vi "APC_9056_DynoControl.vi"(1 "LoadIni?":bool, 2 "PC_ControlSettings":T1={"Spark advance [CADBTDC]"=0.0, "Pref"=0.0, "O2ref"=0.0, "DI advance [CADBTDC]"=0.0, "DI duration [ms] "=0.0, "CO2ref"=0.0, "PFI duration [ms]"=0.0, "IMEP ref"=0.0, "Speed ref"=0.0, "IGN enable"=TRUE, "DI enable"=TRUE, "CL PFI\n lambda"=TRUE, "CL PFI\nIMEP"=FALSE, "Activate\ncylinder"=[FALSE, FALSE, FALSE, FALSE, FALSE, FALSE], "Force idling"=FALSE, "Force motoring"=FALSE, "ETP resync"=FALSE, "Requested mode"=0, "Clear Sync Errors"=FALSE, "toggle TDC"=FALSE, "l ref"=0.0, "PID control references"={"NG"=FALSE, "Ar"=FALSE, "O2"=FALSE, "Intake vent"=FALSE, "Cross vent"=FALSE, "Exhaust vent"=FALSE, "NG control mode"=0, "NG-FC-001-REF"=0.0, "WF-OA-002-REF"=0.0, "IMEP-REF"=0.0, "Nm-REF"=0.0, "Ar control mode"=0, "AR-PC-002-REF"=0.0, "WF-PT-004-REF"=0.0, "O2 control mode"=0, "O2-FC-001-REF"=0.0, "WF-OA-001-REF"=0.0, "Tcoolant control  mode"=0, "EC-FC-001-REF"=0.0, "EC-TT-001-REF"=0.0, "Texh control mode"=0, "SW-FC-004-REF"=0.0, "SW-FT-002-REF"=0.0, "WF-TT-004-REF"=0.0, "Toil control mode"=0, "SW-FC-009-REF"=0.0, "SW-FT-004-REF"=0.0, "EO-TT-001-REF"=0.0, "AIC201_CO2_ConcTarget"=0.0, "O2_FF_NG"=FALSE, "Dyno control mode"=0, "Membrane control mode"=0, "AR-FT-001-REF"=0.0, "MTR modbus floats"=[0.0, 0.0, 0.0, 0.0, 0.0, 0.0, 0.0, 0.0, 0.0, 0.0, 0.0, 0.0, 0.0, 0.0, 0.0, 0.0, 0.0, 0.0, 0.0], "MTR modbus u16"=[0, 0, 0, 0, 0, 0, 0], "MTR HB"=FALSE, "PC_HB"=FALSE, "EMERGENCY STOP"=FALSE}, "CA50setpoint [CADATDC]"=0.0, "CA50 control"=TRUE, "Knock control"=TRUE, "CLEAR EMERGENCY STOP"=FALSE, "EMERGENCY STOP"=FALSE}, 3 "input cluster":T3) -> (0 "DYNO-REF":dbl format="%.2f")   [LabVIEW 2020]
uses:
  controls/APC_PIDCluster.ctl
  controls/APC_ControlSettings.ctl
  controls/APC_PIDcontrolSettings.ctl
  controls/APC_cascadePIDsettings.ctl
  <vilib>/addons/control/pid/pid.llb/PID Advanced (DBL).vi
  <vilib>/Utility/xml.llb/Read From XML File(string).vi
  <vilib>/Utility/xml.llb/Write to XML File(string).vi
  <vilib>/addons/control/pid/NI_PID_pid.lvlib
panel:
  out "direct?":bool
  out "Direct control":dbl format="%.2f"
  in  "SpeedReference (manual)":dbl
  in  "save":bool
  in  "load":bool
  out "Dyno control mode":u8
  out "EngineSpeed":dbl=2293.506542256783
  in  "FF control":dbl format="%.2f"
  in  "reinitialize? (F)":bool
  in  "SpeedSetpointForPID (manual)":dbl
  in  "Dyno control mode":u8=1
  in  "PID gains":T4={"proportional gain (Kc)"=1.0, "integral time (Ti, min)"=0.01, "derivative time (Td, min)"=0.0} {"derivative time (Td, min)" format="%.3f"; "integral time (Ti, min)" format="%.3f"; "proportional gain (Kc)" format="%.3f"}
  in  "PID setpoint range":cluster{"setpoint high":dbl, "setpoint low":dbl}={"setpoint high"=100.0, "setpoint low"=0.0} {"setpoint high" format="%.2f"; "setpoint low" format="%.2f"}
  in  "PID output range":cluster{"output high":dbl, "output low":dbl}={"output high"=100.0, "output low"=-100.0} {"output low" format="%.2f"; "output high" format="%.2f"}
  in  "Override PC PID references":bool
  in  "Safe mode control":dbl format="%.2f"
  in  "learn?":bool
  out "CL on?":bool
  out "setpoint":dbl format="%.2f"
  # "Dyno control"
  # "Modes:\n0 : safe. 0 sent to dyno\n1 (default) : speed reference sent to dyno\n2 : a PID correction is added to the direct control. Tune the parameters with care (mostly slow integral action, no proportional or feed forward)"
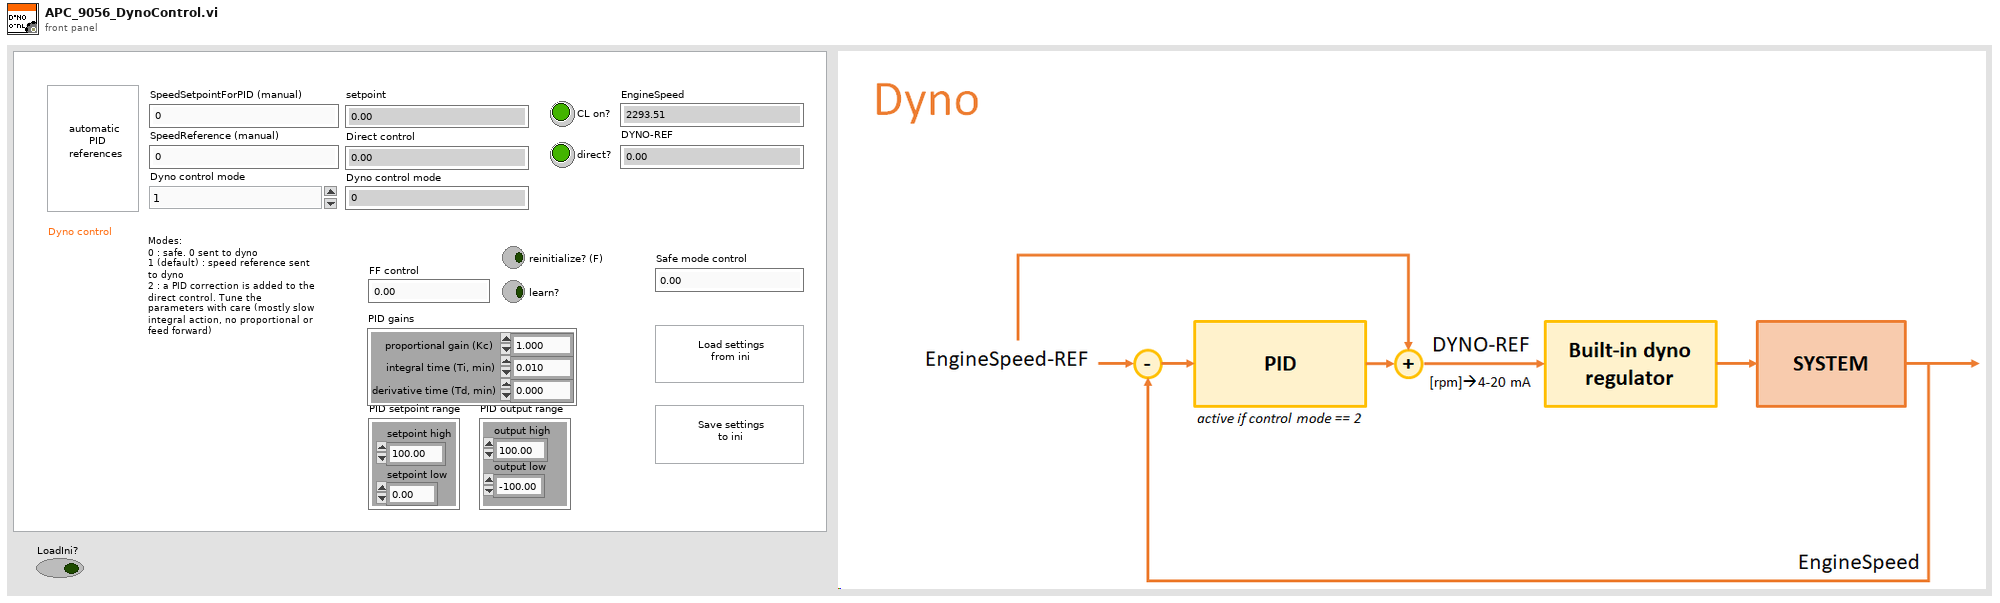
[diagram p1: front panel]
types:
  T1 = typedef "APC_ControlSettings.ctl" = cluster{"Spark advance [CADBTDC]":dbl, "Pref":dbl, "O2ref":dbl, "DI advance [CADBTDC]":dbl, "DI duration [ms] ":dbl, "CO2ref":dbl, "PFI duration [ms]":dbl, "IMEP ref":dbl, "Speed ref":dbl, "IGN enable":bool, "DI enable":bool, "CL PFI\n lambda":bool, "CL PFI\nIMEP":bool, "Activate\ncylinder":bool[], "Force idling":bool, "Force motoring":bool, "ETP resync":bool, "Requested mode":i8, "Clear Sync Errors":bool, "toggle TDC":bool, "l ref":dbl, "PID control references":T2, "CA50setpoint [CADATDC]":dbl, "CA50 control":bool, "Knock control":bool, "CLEAR EMERGENCY STOP":bool, "EMERGENCY STOP":bool}
  T2 = typedef "APC_PIDcontrolSettings.ctl" = cluster{"NG":bool, "Ar":bool, "O2":bool, "Intake vent":bool, "Cross vent":bool, "Exhaust vent":bool, "NG control mode":u8, "NG-FC-001-REF":dbl, "WF-OA-002-REF":dbl, "IMEP-REF":dbl, "Nm-REF":dbl, "Ar control mode":u8, "AR-PC-002-REF":dbl, "WF-PT-004-REF":dbl, "O2 control mode":u8, "O2-FC-001-REF":dbl, "WF-OA-001-REF":dbl, "Tcoolant control  mode":u8, "EC-FC-001-REF":dbl, "EC-TT-001-REF":dbl, "Texh control mode":u8, "SW-FC-004-REF":dbl, "SW-FT-002-REF":dbl, "WF-TT-004-REF":dbl, "Toil control mode":u8, "SW-FC-009-REF":dbl, "SW-FT-004-REF":dbl, "EO-TT-001-REF":dbl, "AIC201_CO2_ConcTarget":dbl, "O2_FF_NG":bool, "Dyno control mode":u8, "Membrane control mode":u8, "AR-FT-001-REF":dbl, "MTR modbus floats":sgl[], "MTR modbus u16":u16[], "MTR HB":bool, "PC_HB":bool, "EMERGENCY STOP":bool}
  T3 = typedef "APC_PIDCluster.ctl" = cluster{"AR-FT-001":dbl, "O2-FC-001":dbl, "SW-FT-004":dbl, "SW-FT-002":dbl, "WF-OA-002":dbl, "WF-PT-004":dbl, "WF-OA-001":dbl, "EC-TT-001":dbl, "WF-TT-004":dbl, "EC-FC-001":dbl, "NG-FC-001":dbl, "EO-TT-001":dbl, "SW-FC-008":dbl, "SW-FC-004":dbl, "IMEPn6":dbl, "TORQUE":dbl, "CylPresWarnings":dbl, "CylPresErrors":dbl, "NG-FT-001":dbl, "EngineSpeed_rpm":dbl}
  T4 = cluster{"proportional gain (Kc)":dbl, "integral time (Ti, min)":dbl, "derivative time (Td, min)":dbl}
  T5 = typedef "APC_cascadePIDsettings.ctl" = cluster{"HL FF control":dbl, "LL FF control":dbl, "HL PID gains":cluster{"proportional gain (Kc)":dbl, "integral time (Ti, min)":dbl, "derivative time (Td, min)":dbl}, "LL PID gains":cluster{"proportional gain (Kc)":dbl, "integral time (Ti, min)":dbl, "derivative time (Td, min)":dbl}, "HL PID setpoint range":cluster{"setpoint high":dbl, "setpoint low":dbl}, "HL PID output range":cluster{"output high":dbl, "output low":dbl}, "LL PID setpoint range":cluster{"setpoint high":dbl, "setpoint low":dbl}, "LL PID output range":cluster{"output high":dbl, "output low":dbl}, "Safe mode control":dbl}
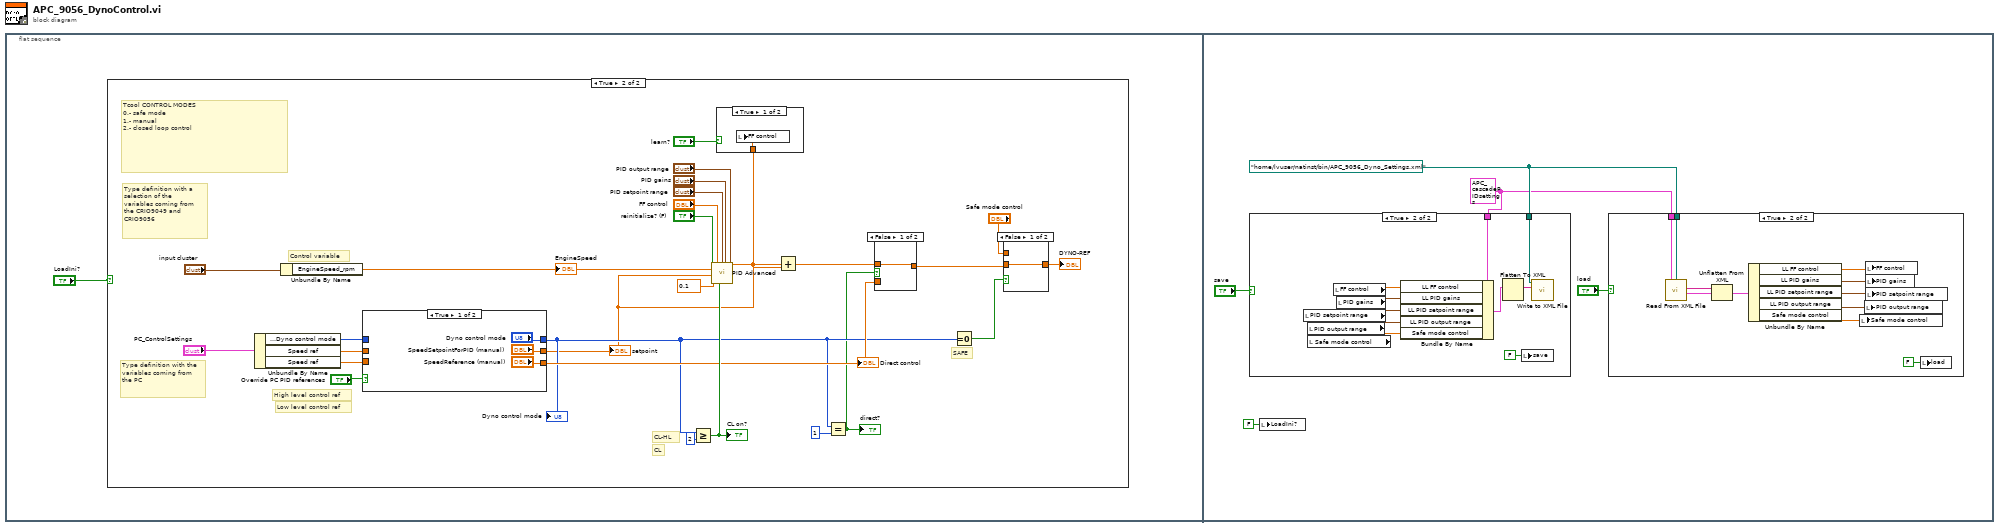
[diagram p0: block diagram]
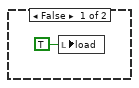
[diagram p2: hidden frame]
diagram:
  n1 = flat-sequence {
    frame #0 {
      n2 = case shown="True" "LoadIni?" {
        frame False {
          n3 = local write "load"(TRUE ("load")) -> ()
        }
        frame True {
          # "Type definition with a selection of the variables coming from the CRIO9049 and CRIO9056"
          # "Type definition with the variables coming from the PC"
          # "Low level control ref"
          # "High level control ref"
          # "Control variable"
          # "SAFE"
          # "CL-HL"
          # "CL"
          # "Tcool CONTROL MODES\n0.- safe mode\n1.- manual\n2.- closed loop control"
          n4 = Unbundle By Name("PC_ControlSettings") -> ("PID control references.Dyno control mode"=w3:u8, "Speed ref"=w17:dbl, "Speed ref"=w12:dbl)
          n5 = Unbundle By Name("input cluster") -> ("EngineSpeed_rpm"=w15:dbl)
          "EngineSpeed" <- w15
          n6 = case shown="True" "Override PC PID references" {
            tunnel: w17 -> [_ w40]
            tunnel: ["Dyno control mode" w38] -> w8
            tunnel: ["SpeedSetpointForPID (manual)" w40] -> w4
            tunnel: ["SpeedReference (manual)" w39] -> w9
            tunnel: w12 -> [_ w39]
            tunnel: w3 -> [_ w38]
            frame True {
            }
            frame False {
            }
          }
          "setpoint" <- w4
          "Dyno control mode" <- w8
          "Direct control" <- w9
          n7 = Greater Or Equal?(x=w8, y=u8 2) -> (x >= y?=w27:bool)
          "CL on?" <- w27
          n8 = call-poly <vilib>:"PID Advanced.vi"("setpoint"=w4, "output range"="PID output range", "auto? (T)"=w27, "manual control"="FF control", "process variable"=w15, "setpoint range"="PID setpoint range", "PID gains"="PID gains", "dt (s)"=0.1, "reinitialize? (F)"="reinitialize? (F)") -> ("output"=w6:dbl)  [unwired: 5 in, 1 out]
          n9 = case shown="True" "learn?" {
            tunnel: w6 -> [w32 _]
            frame True {
              n10 = local write "FF control"(w32) -> ()
            }
            frame False {
            }
          }
          n11 = Add(x=w6, y=w4) -> (x+y=w5:dbl)
          n12 = Equal?(x=w8, y=u8 1) -> (x = y?=w7:bool)
          "direct?" <- w7
          n13 = case shown="False" w7 {
            tunnel: [w30 w31] -> w10
            tunnel: w5 -> [w30 _]
            tunnel: w9 -> [_ w31]
            frame False {
            }
            frame True {
            }
          }
          n14 = Equal To 0?(x=w8) -> (x = 0?=w29:bool)
          n15 = case shown="False" w29 {
            tunnel: [w33 w34] -> w23
            tunnel: "Safe mode control" -> [_ w34]
            tunnel: w10 -> [w33 _]
            frame False {
            }
            frame True {
            }
          }
          "DYNO-REF" <- w23
        }
      }
    }
    frame #1 {
      w43 = path "/home/lvuser/natinst/bin/APC_9056_Dyno_Settings.xml" ("XML File Path")
      w42 = T5 {"HL FF control"=0.0, "LL FF control"=0.0, "HL PID gains"={"proportional gain (Kc)"=1.0, "integral time (Ti, min)"=0.01, "derivative time (Td, min)"=0.0}, "LL PID gains"={"proportional gain (Kc)"=1.0, "integral time (Ti, min)"=0.01, "derivative time (Td, min)"=0.0}, "HL PID setpoint range"={"setpoint high"=100.0, "setpoint low"=0.0}, "HL PID output range"={"output high"=0.0, "output low"=0.0}, "LL PID setpoint range"={"setpoint high"=100.0, "setpoint low"=0.0}, "LL PID output range"={"output high"=10.0, "output low"=-10.0}, "Safe mode control"=0.0} ("Cluster")
      n16 = case shown="True" "save" {
        tunnel: w43 -> [_ w58]
        tunnel: w42 -> [_ w57]
        frame False {
        }
        frame True {
          n17 = local read "PID setpoint range"() -> (w63:cluster{"setpoint high":dbl, "setpoint low":dbl})
          n18 = local read "PID output range"() -> (w62:cluster{"output high":dbl, "output low":dbl})
          n19 = local read "Safe mode control"() -> (w61:dbl)
          n20 = local read "FF control"() -> (w65:dbl)
          n21 = local read "PID gains"() -> (w64:T4)
          n22 = Bundle By Name(cluster=w57, "LL FF control"=w65, "LL PID gains"=w64, "LL PID setpoint range"=w63, "LL PID output range"=w62, "Safe mode control"=w61) -> (w60:T5)
          n23 = Flatten To XML(6:w60) -> (2:w59:string)
          n24 = local write "save"(FALSE ("load")) -> ()
          n25 = call-poly <vilib>:"Write to XML File.vi"("XML Input"=w59, "XML File Path"=w58) -> ()  [unwired: 7 in, 3 out]
        }
      }
      n26 = local write "LoadIni?"(FALSE ("LoadIni?")) -> ()
      n27 = case shown="True" "load" {
        tunnel: w43 -> [_ w54]
        tunnel: w42 -> [_ w53]
        frame False {
        }
        frame True {
          n28 = call-poly <vilib>:"Read From XML File.vi"("XML File Path"=w54) -> ("XML Elements"=w55:string)  [unwired: 8 in, 2 out]
          n29 = Unflatten From XML(xml string=w55, type=w53) -> (value=w52:T5)  [unwired: 1 in, 1 out]
          n30 = Unbundle By Name(w52) -> ("LL FF control"=w51:dbl, "LL PID gains"=w50:T4, "LL PID setpoint range"=w49:cluster{"setpoint high":dbl, "setpoint low":dbl}, "LL PID output range"=w48:cluster{"output high":dbl, "output low":dbl}, "Safe mode control"=w47:dbl)
          n31 = local write "Safe mode control"(w47) -> ()
          n32 = local write "PID output range"(w48) -> ()
          n33 = local write "FF control"(w51) -> ()
          n34 = local write "PID gains"(w50) -> ()
          n35 = local write "PID setpoint range"(w49) -> ()
          n36 = local write "load"(FALSE ("save")) -> ()
        }
      }
    }
  }
